vi "MSEditor SubVI MathieuEqCalculator.vi"(1 "Target (Freq)":enum16{"m/z", "Volt", "Freq", "Beta"}(ring)=enum."Freq", 3 "Parametres in":T1={"mz(Th)"=0.0, "Amp(V)"=330.0, "Freq(Hz)"=0.0, "Beta"=1.0, "r_0 (mm)"=10.0, "z_0 (mm)"=7.0710678118654755}) -> (0 "Parametres out":T1)   [LabVIEW 2018]
uses:
  PublicSubVI/Ctl/MathieuEqParam.ctl
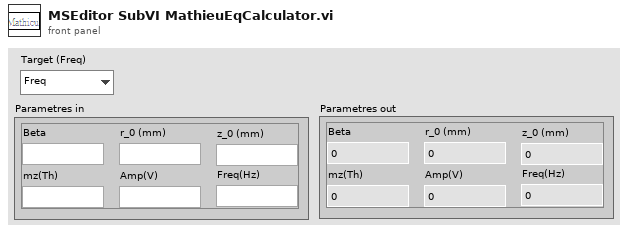
[diagram p1: front panel]
types:
  T1 = typedef "MathieuEqParam.ctl" = cluster{"mz(Th)":ext, "Amp(V)":ext, "Freq(Hz)":ext, "Beta":ext, "r_0 (mm)":ext, "z_0 (mm)":ext}
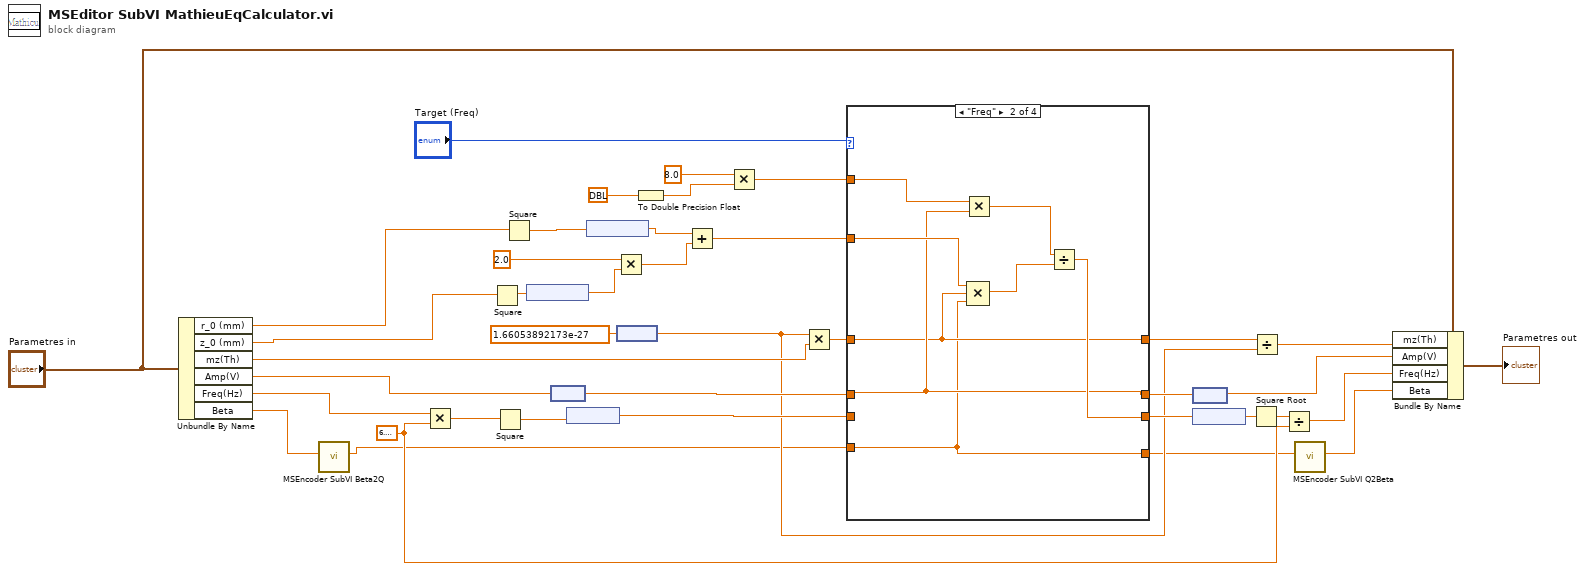
[diagram p0: block diagram]
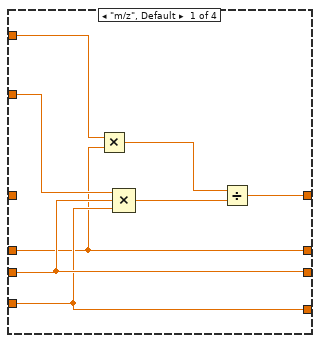
[diagram p2: hidden frame]
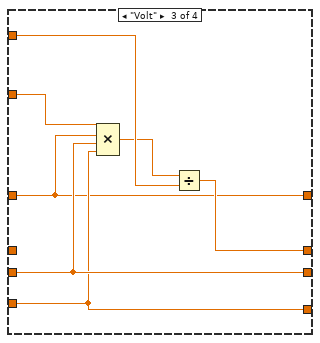
[diagram p3: hidden frame]
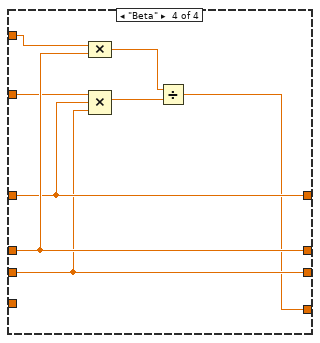
[diagram p4: hidden frame]
diagram:
  w14 = 6.283185307179586
  n1 = Unbundle By Name("Parametres in") -> ("r_0 (mm)"=w9:ext, "z_0 (mm)"=w8:ext, "mz(Th)"=w33:ext, "Amp(V)"=w23:ext, "Freq(Hz)"=w24:ext, "Beta"=w5:ext)
  n2 = call "MSEncoder SubVI Beta2Q.vi"("Beta"=w5) -> ("Q"=w4:dbl)  [unwired: 10 in]
  n3 = Multiply(x=w24, y=w14) -> (x*y=w31:ext)
  n4 = Square(x=w8) -> (x^2=w10:ext)
  n5 = Square(x=w31) -> (x^2=w26:ext)
  n6 = Square(x=w9) -> (x^2=w29:ext)
  n7 = node(w10) -> (w27:ext[unit])
  n8 = node(w23) -> (w22:ext[unit])
  n9 = node(w26) -> (w25:ext[unit])
  n10 = node(w29) -> (w28:ext[unit])
  n11 = Multiply(x=2.0, y=w27) -> (x*y=w38:ext[unit])
  n12 = node(1.66053892173e-27) -> (w16:dbl[unit])
  n13 = To Double Precision Float(number=ext[unit] 1.6021766208e-19) -> (double precision float=w35:dbl[unit])
  n14 = Add(x=w28, y=w38) -> (x+y=w7:ext[unit])
  n15 = Multiply(x=8.0, y=w35) -> (x*y=w30:dbl[unit])
  n16 = Multiply(x=w16, y=w33) -> (x*y=w32:ext[unit])
  n17 = case shown="\"Freq\"" "Target (Freq)" {
    tunnel: w32 -> [_ w49 w56 w67]
    tunnel: w4 -> [w41 w48 w57 _]
    tunnel: w30 -> [w47 w55 w62 w70]
    tunnel: w7 -> [w46 w54 w61 w68]
    tunnel: w25 -> [w42 _ w58 w66]
    tunnel: w22 -> [w40 w50 _ w69]
    tunnel: [w40 w50 w59 w69] -> w21
    tunnel: [w42 w51 w58 w66] -> w20
    tunnel: [w41 w48 w57 w63] -> w3
    tunnel: [w43 w49 w56 w67] -> w17
    frame "m/z", Default {
      n18 = Multiply(x=w47, y=w40) -> (x*y=w45:ext[unit])
      n19 = Compound Arithmetic op=MULTIPLY(w46, w42, w41) -> (w44:ext[unit])
      n20 = Divide(x=w45, y=w44) -> (x/y=w43:ext[unit])
    }
    frame "Freq" {
      n21 = Multiply(x=w55, y=w50) -> (x*y=w53:ext[unit])
      n22 = Compound Arithmetic op=MULTIPLY(w54, w49, w48) -> (w52:ext[unit])
      n23 = Divide(x=w53, y=w52) -> (x/y=w51:ext[unit])
    }
    frame "Volt" {
      n24 = Compound Arithmetic op=MULTIPLY(w61, w56, w58, w57) -> (w60:ext[unit])
      n25 = Divide(x=w60, y=w62) -> (x/y=w59:ext[unit])
    }
    frame "Beta" {
      n26 = Compound Arithmetic op=MULTIPLY(w70, w69) -> (w64:ext[unit])
      n27 = Compound Arithmetic op=MULTIPLY(w68, w67, w66) -> (w65:ext[unit])
      n28 = Divide(x=w64, y=w65) -> (x/y=w63:ext)
    }
  }
  n29 = node(w21) -> (w12:ext)
  n30 = node(w20) -> (w19:ext)
  n31 = Square Root(x=w19) -> (sqrt(x)=w15:ext)
  n32 = Divide(x=w17, y=w16) -> (x/y=w13:ext)
  n33 = Divide(x=w15, y=w14) -> (x/y=w11:ext)
  n34 = call "MSEncoder SubVI Q2Beta.vi"("q_z"=w3) -> ("Beta"=w2:dbl)  [unwired: 10 in]
  n35 = Bundle By Name(cluster="Parametres in", "mz(Th)"=w13, "Amp(V)"=w12, "Freq(Hz)"=w11, "Beta"=w2) -> (→"Parametres out":T1)
